vi "ScaleSineWaveParams.vi"(8 "error in (no error)":errorcluster, 9 "FPGA Clock Rate":dbl=40000000.0, 10 "max voltage for target":dbl=5.0, 11 "Sine wave":T1) -> (0 "error out":errorcluster, 3 "Sinewave Props":T2)   [LabVIEW 2021]
uses:
  <vilib>/rvi/Analysis/host/Public/NI_FpgaMspHost.lvlib
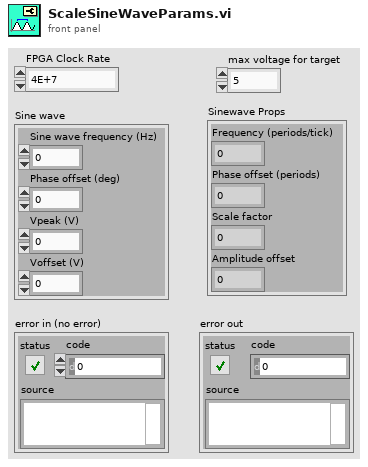
[diagram p1: front panel]
types:
  T1 = cluster{"Sine wave frequency (Hz)":dbl, "Phase offset (deg)":dbl, "Vpeak (V)":dbl, "Voffset (V)":dbl}
  T2 = cluster{"Frequency (periods/tick)":fxp<+,32,0>, "Phase offset (periods)":fxp<+,32,0>, "Scale factor":fxp<+,12,1>, "Amplitude offset":fxp<+/-,16,12>}
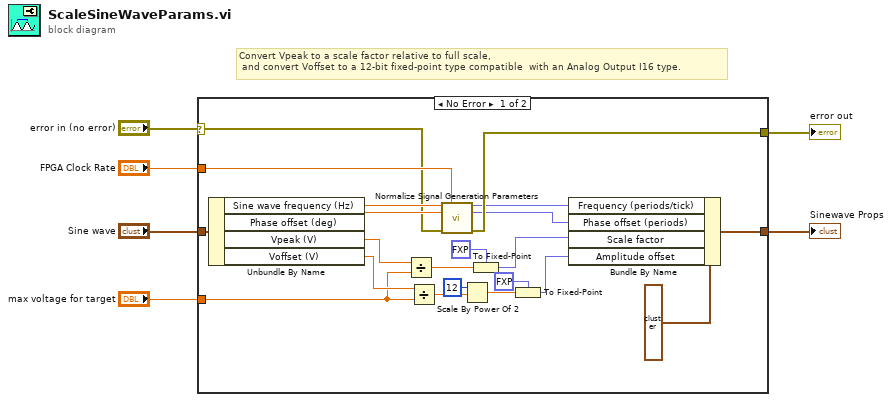
[diagram p0: block diagram]
diagram:
  # "Convert Vpeak to a scale factor relative to full scale,\n and convert Voffset to a 12-bit fixed-point type compatible  with an Analog Output I16 type."
  n1 = case shown="No Error" "error in (no error)" {
    selector: "error in (no error)" -> [w7 _]
    tunnel: [w27 _] -> w6
    tunnel: [w26 _] -> w5
    tunnel: "Sine wave" -> [w15 _]
    tunnel: "FPGA Clock Rate" -> [w14 _]
    tunnel: "max voltage for target" -> [w11 _]
    frame No Error {
      n2 = Unbundle By Name(w15) -> ("Sine wave frequency (Hz)"=w12:dbl, "Phase offset (deg)"=w13:dbl, "Vpeak (V)"=w16:dbl, "Voffset (V)"=w17:dbl)
      n3 = Divide(x=w16, y=w11) -> (x/y=w18:dbl)
      n4 = Divide(x=w17, y=w11) -> (x/y=w10:dbl)
      n5 = call <vilib>:"Normalize Signal Generation Parameters.vi"("frequency (Hz)"=w12, "FPGA clock rate (Hz)"=w14, "phase offset (deg)"=w13, "error in (no error)"=w7) -> ("frequency (periods/tick)"=w21:fxp<+,32,0>, "phase offset (periods)"=w22:fxp<+,32,0>, "error out"=w26:errorcluster)  [unwired: 6 in, 3 out]
      n6 = Scale By Power Of 2(n=i16 12, x=w10) -> (x*2^n=w8:dbl)
      n7 = To Fixed-Point(fixed-point type=fxp<+,12,1> 1.0 ("Scale factor"), number=w18) -> (fixed-point=w23:fxp<+,12,1>)
      n8 = To Fixed-Point(fixed-point type=fxp<+/-,16,12> 0.0 ("Amplitude offset"), number=w8) -> (fixed-point=w24:fxp<+/-,16,12>)
      n9 = Bundle By Name(cluster=T2 {"Frequency (periods/tick)"=0.0, "Phase offset (periods)"=0.0, "Scale factor"=1.0, "Amplitude offset"=0.0} ("Sinewave Props 0"), "Frequency (periods/tick)"=w21, "Phase offset (periods)"=w22, "Scale factor"=w23, "Amplitude offset"=w24) -> (w27:T2)
    }
    frame Error {
    }
  }
  "Sinewave Props" <- w6
  "error out" <- w5
